vi "Que_elements_GCFS.vi"(5 "Pixel values":string[][](array[string]), 6 "queue":refnum<queue>, 7 "Freezing points":string[][](array[string]), 8 "error in (no error)":errorcluster, 9 "Snap timestamp":string, 10 "Image To Save":T1, 11 "FreezingData":bool) -> (0 "error out":errorcluster, 1 "timed out?":bool, 3 "queue out":refnum<queue>)   [LabVIEW 2024]
uses:
  <vilib>/vision/Image Controls.llb/IMAQ Image.ctl
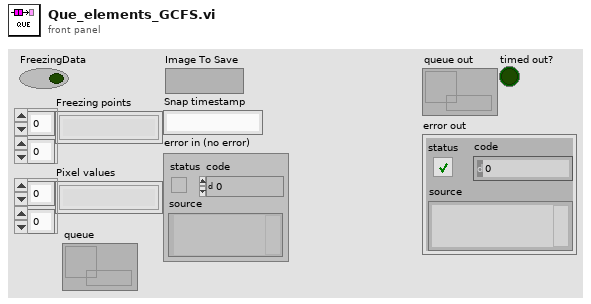
[diagram p1: front panel]
types:
  T1 = typedef "IMAQ Image.ctl" = refnum<image>
  T2 = cluster{"Image To Save":T1, "Snap timestamp":string, "Pixel values":string[][], "Freezing points":string[][], "FreezingData":bool, "Image Pixels (U16)":u16[][]}
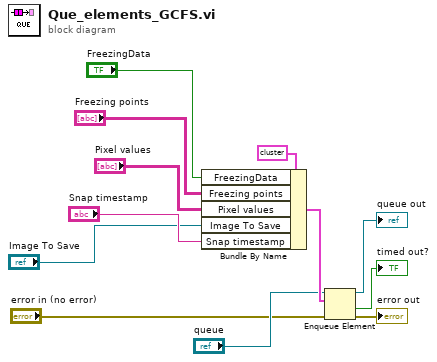
[diagram p0: block diagram]
diagram:
  n1 = Bundle By Name(cluster=T2 {"Image To Save"=refnum, "Snap timestamp"="", "Pixel values"=[], "Freezing points"=[], "FreezingData"=FALSE, "Image Pixels (U16)"=[]}, "FreezingData"="FreezingData", "Freezing points"="Freezing points", "Pixel values"="Pixel values", "Image To Save"="Image To Save", "Snap timestamp"="Snap timestamp") -> (w12:T2)
  n2 = Enqueue Element(queue="queue", element=w12, error in (no error)="error in (no error)") -> (queue out=→"queue out":refnum<queue>, timed out?=→"timed out?":bool, error out=→"error out":errorcluster)  [unwired: 1 in]
